vi "Load Instrument Classes.vi"(8 "error in (no error)":errorcluster, 11 "C.E.":refnum<class "Control Experiment.lvclass">) -> (0 "error out":errorcluster, 3 "Control Experiment":refnum<class "Control Experiment.lvclass">)   [LabVIEW 2019, in "Control Experiment.lvclass"]
uses:
  Control Experiment.lvclass
  Typedefs/Instrument Class Rings--Cluster.ctl
  <userlib>/LevyLab/Instrument Framework/Instrument/Instrument.lvclass
  C:/Program Files (x86)/National Instruments/LabVIEW 2019/vi.lib/JKI/JKI SMO/SMO/SMO.lvclass
  Control Experiment.lvclass/Control Experiment.ctl
  Typedefs/Instrument Classes--cluster.ctl
  <userlib>/LevyLab/Instrument Framework/Instrument Types/Lockin/Instrument.LockinAPI.lvclass
  <userlib>/LevyLab/Instrument Framework/Instrument Types/Amplifier/Instrument.Amplifier.lvclass
  <userlib>/LevyLab/Instrument Framework/Instrument Types/Cryostat/Instrument.Cryostat.lvclass
  <userlib>/LevyLab/Instrument Framework/Instrument Types/CBridge/Instrument.CBridge.lvclass
  <userlib>/LevyLab/Instrument Framework/Instrument Types/Delay Line/Instrument.DelayLine.lvclass
  <userlib>/LevyLab/Instrument Framework/Instrument Types/Strain/Instrument.Strain.lvclass
  <userlib>/LevyLab/Instrument Framework/Instrument Types/VNA/Instrument.VNA.lvclass
  <userlib>/LevyLab/Instrument Framework/Instrument Types/VSource/Instrument.VSource.lvclass
  Typedefs/Instrument Types--enum.ctl
  <userlib>/LevyLab/Instrument Framework/Instrument/Instrument.lvclass/Instrument.ctl
  <vilib>/Utility/Data Type/NI_Data Type.lvlib
  Attributes/Instrument Attributes.lvlib
  <vilib>/JKI/JKI SMO/URI Parsing/URI.lvlib
panel:
  in  "DAQ":refnum<visa-resource-name>
  in  "Instrument Addresses":T1 caption="Instruments"
  in  "OK":bool
  in  "Instrument Classes":T2 {"Amplifier" items=["", "Krohn-Hite-7008"]; "DAQ" items=["", "Lockin"]; "Strain Cell" items=["", "RP100"]; "Capacitance" items=["", "AH2500"]; "Level" items=["", "Cryostation", "OxfordVRM", "OptiCool", "PPMS", "PPMS1", "PPMS2", "PPMS3"]; "Rotator" items=["", "Cryostation", "OxfordVRM", "OptiCool", "PPMS", "PPMS1", "PPMS2", "PPMS3"]; "Magnet" items=["", "Cryostation", "OxfordVRM", "OptiCool", "PPMS", "PPMS1", "PPMS2", "PPMS3"]; "Temperature" items=["", "Cryostation", "OxfordVRM", "OptiCool", "PPMS", "PPMS1", "PPMS2", "PPMS3"]}
  out "Status":string
  # "1. Choose / Confirm Instrument Classes"
  # "2. Choose / Confirm Remote Instruments"
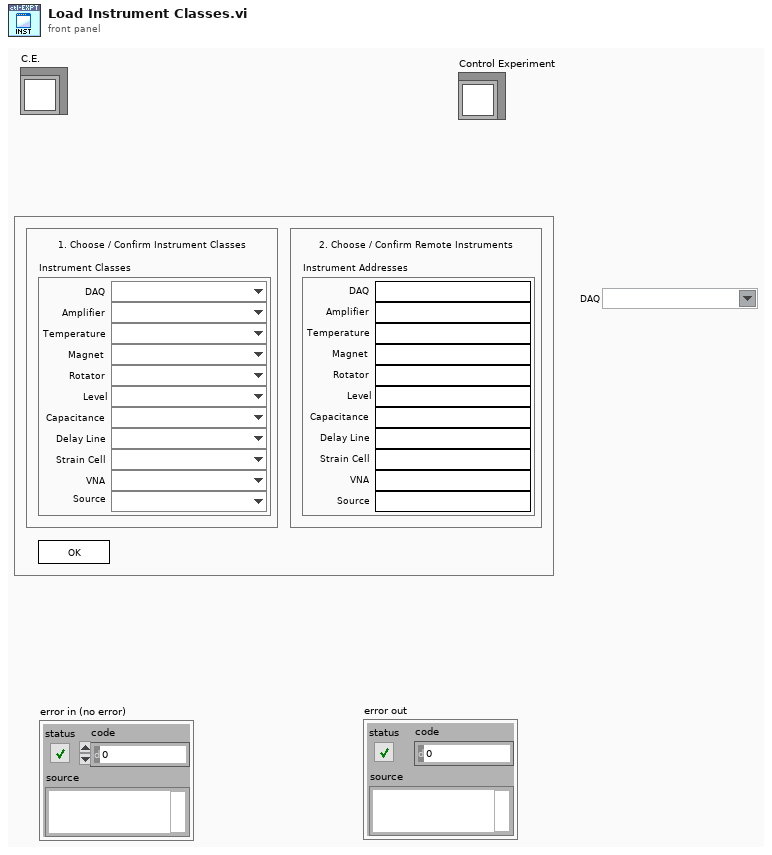
[diagram p1: front panel]
types:
  T1 = cluster{"DAQ":string, "Amplifier":string, "Temperature":string, "Magnet":string, "Rotator":string, "Level":string, "Capacitance Bridge":string, "Delay Line":string, "Strain Cell":string, "VNA":string, "Source":string}
  T2 = typedef "Control Experiment.lvclass/Instrument Class Rings--Cluster.ctl" = cluster{"DAQ":u16, "Amplifier":u16, "Temperature":u16, "Magnet":u16, "Rotator":u16, "Level":u16, "Capacitance":u16, "Delay Line":u16, "Strain Cell":u16, "VNA":u16, "Source":u16}
  T3 = enum32{"Invalid", "Standard", "Closed", "Hidden", "Minimized", "Maximized"}
  T4 = enum32{"invalid app kind", "Development System", "Run Time System", "Student Edition", "Embedded LabVIEW", "Evaluation", "Custom"}
  T5 = typedef "Control Experiment.lvclass/Instrument Classes--cluster.ctl" = cluster{"DAQ":refnum<class "Instrument.LockinAPI.lvclass">, "Amplifier":refnum<class "Instrument.Amplifier.lvclass">, "Temperature":refnum<class "Instrument.Cryostat.lvclass">, "Magnet":refnum<class "Instrument.Cryostat.lvclass">, "Rotator":refnum<class "Instrument.Cryostat.lvclass">, "Level":refnum<class "Instrument.Cryostat.lvclass">, "Capacitance":refnum<class "Instrument.CBridge.lvclass">, "Delay Line":refnum<class "Instrument.DelayLine.lvclass">, "Strain Cell":refnum<class "Instrument.Strain.lvclass">, "VNA":refnum<class "Instrument.VNA.lvclass">, "Source":refnum<class "Instrument.VSource.lvclass">}
  T6 = typedef "Control Experiment.lvclass/Instrument Types--enum.ctl" = enum16{"DAQ", "Amplifier", "Temperature", "Magnet", "Rotator", "Level", "Capacitance", "Delay Line", "Strain Cell", "VNA", "Source"}
  T7 = cluster{"Core":cluster{"Current VI Reference":refnum<vi>, "Close Panel on Exit?":bool}, "C.E.":refnum<class "Control Experiment.lvclass">, "Instruments":refnum<vi>, "Addresses":refnum<vi>, "Instrument Class Rings":refnum<vi>[], "Installed Instruments":refnum<class "Instrument.lvclass">[], "Cast Instruments":refnum<class "Instrument.lvclass">[]}
  T8 = cluster{"Current VI Reference":refnum<vi>, "Close Panel on Exit?":bool}
  T9 = enum32{"Bad", "Idle", "Run top level", "Running"}
  T10 = typedef "Control Experiment.lvclass/Instruments--cluster.ctl" = cluster{"class path":path, "Address":string, "Type":T6}
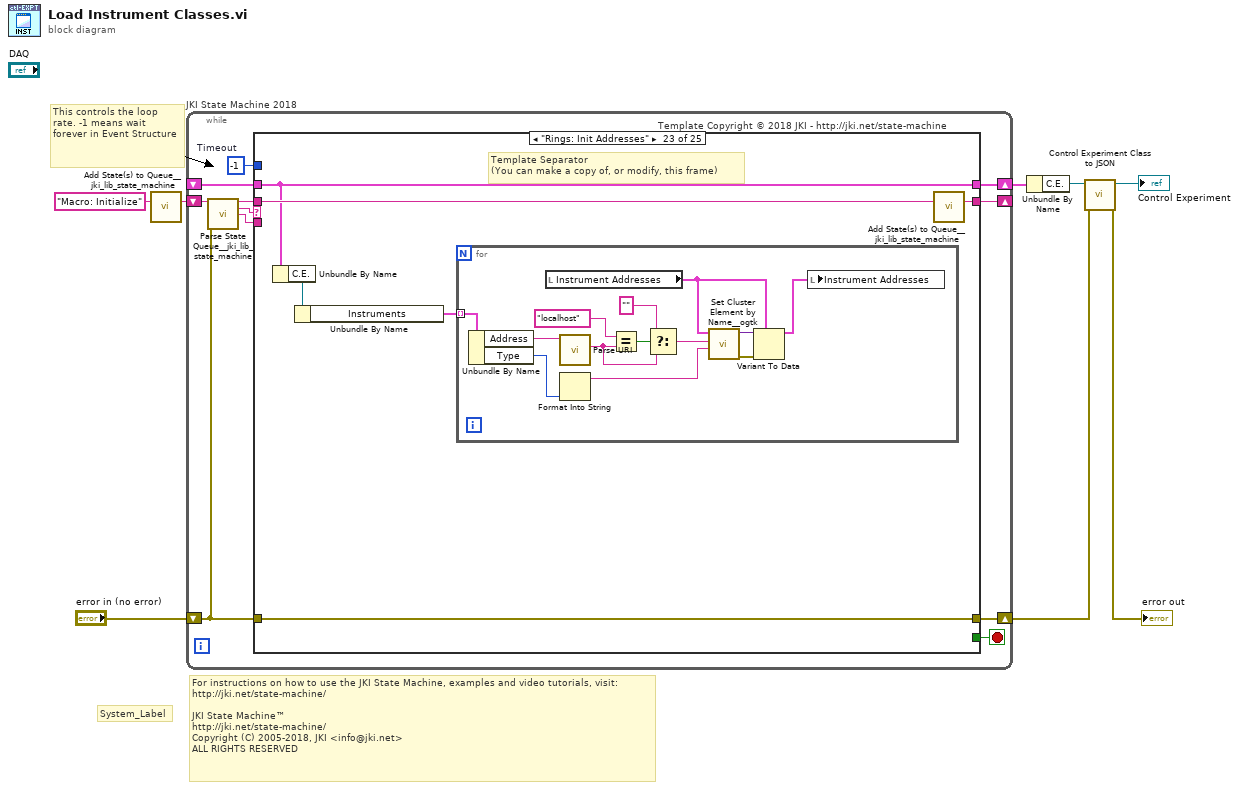
[diagram p0: block diagram]
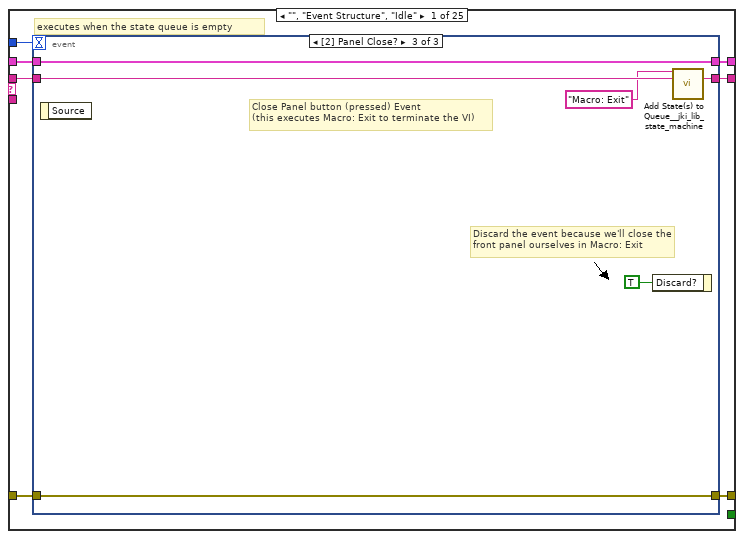
[diagram p2: hidden frame]
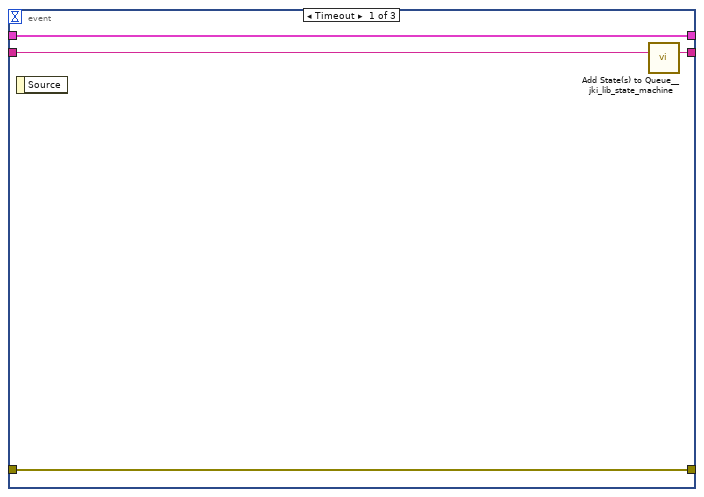
[diagram p3: hidden frame]
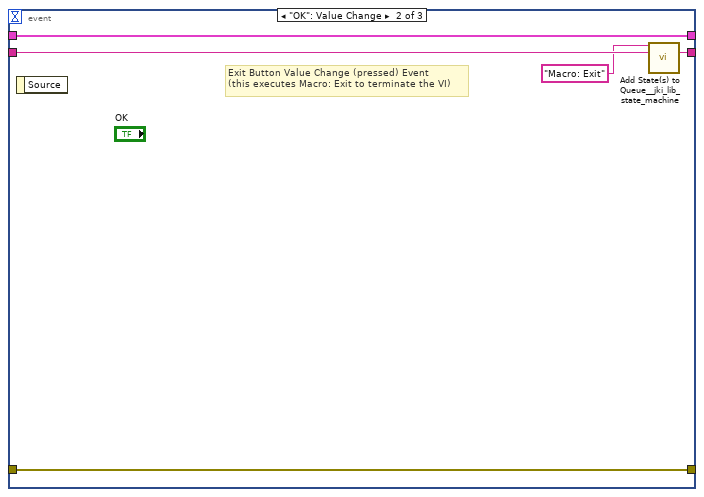
[diagram p4: hidden frame]
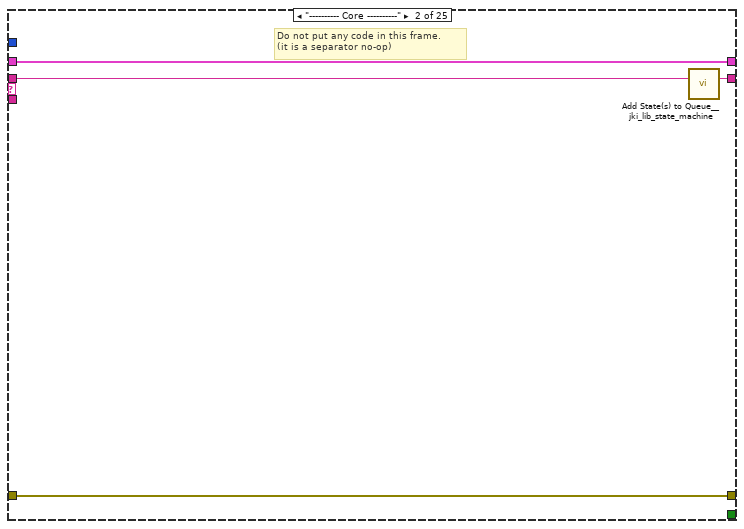
[diagram p5: hidden frame]
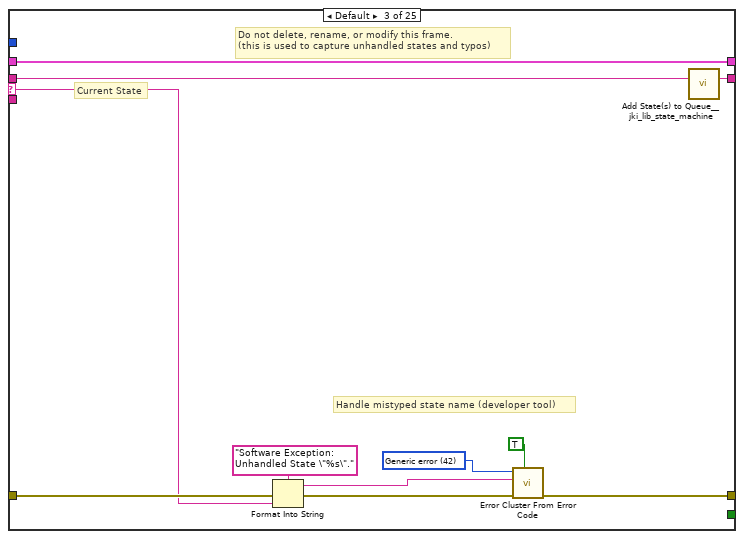
[diagram p6: hidden frame]
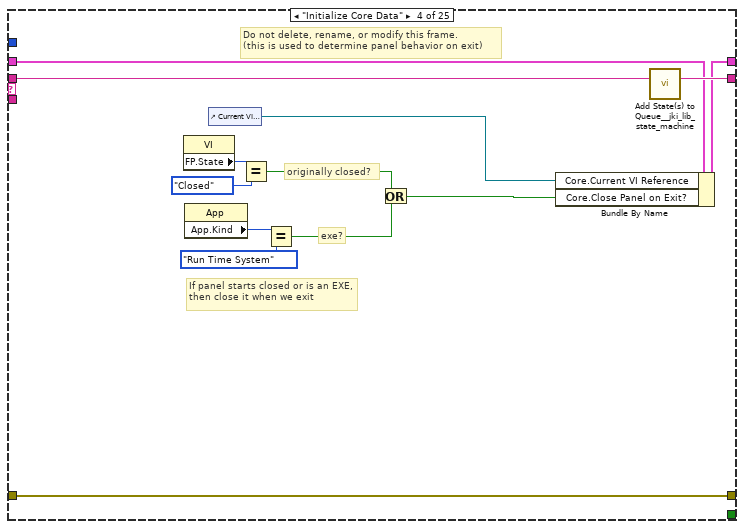
[diagram p7: hidden frame]
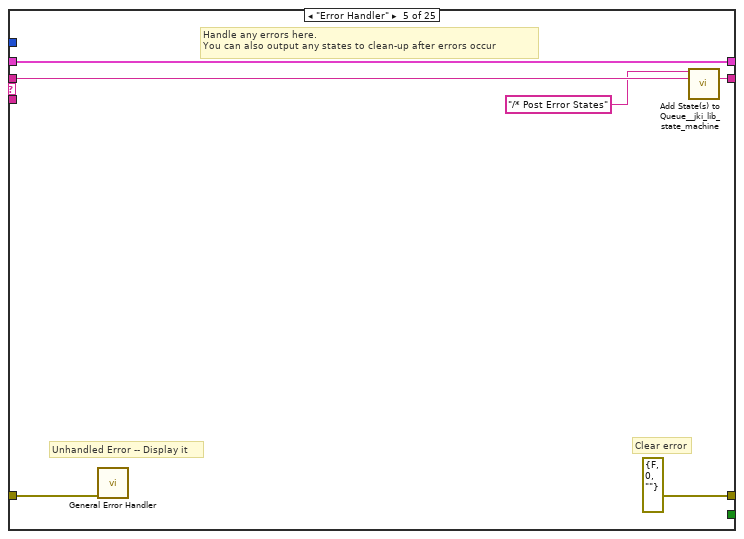
[diagram p8: hidden frame]
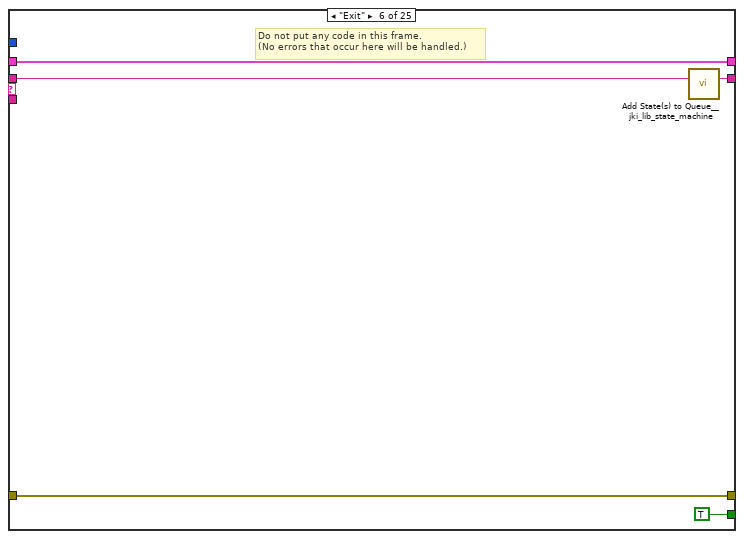
[diagram p9: hidden frame]
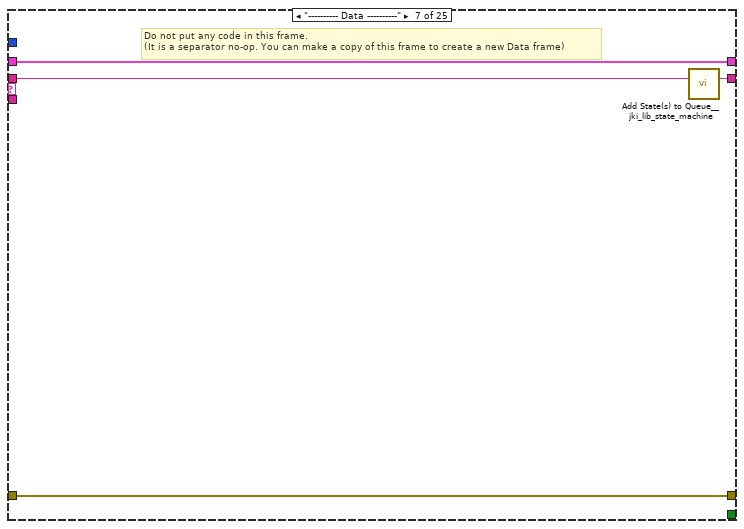
[diagram p10: hidden frame]
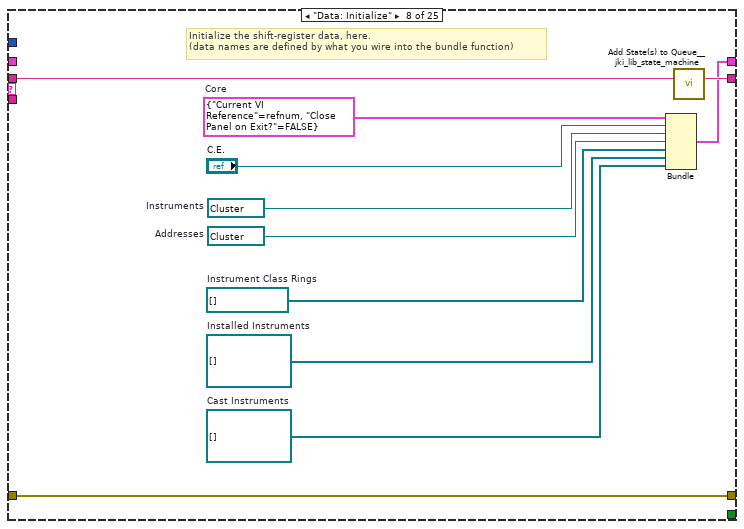
[diagram p11: hidden frame]
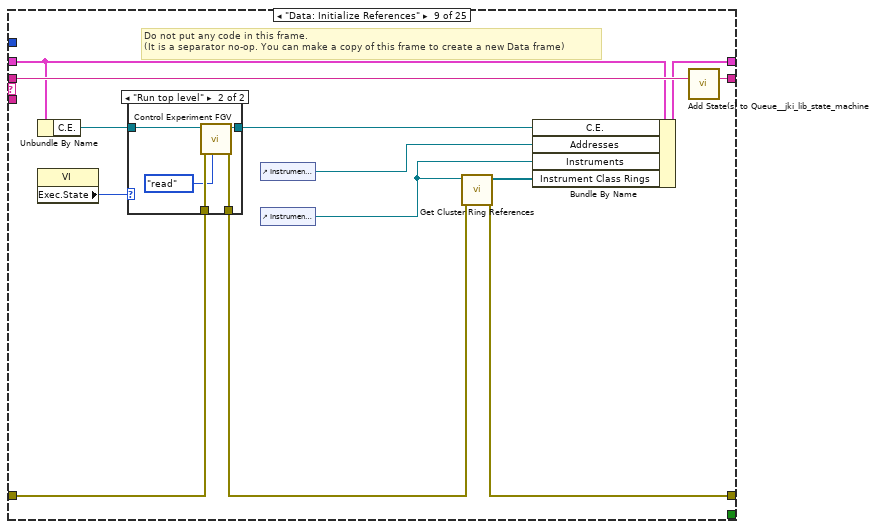
[diagram p12: hidden frame]
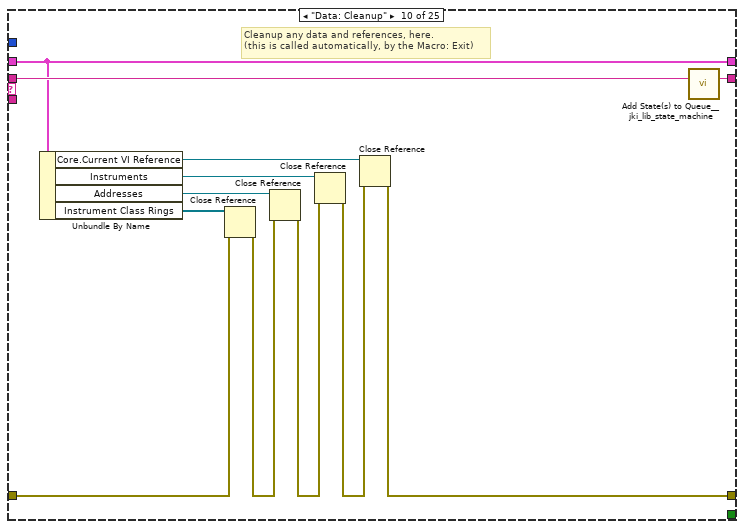
[diagram p14: hidden frame]
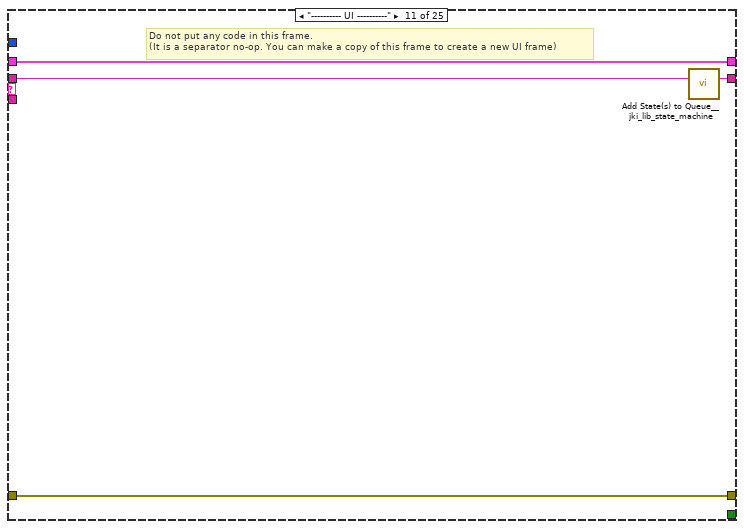
[diagram p15: hidden frame]
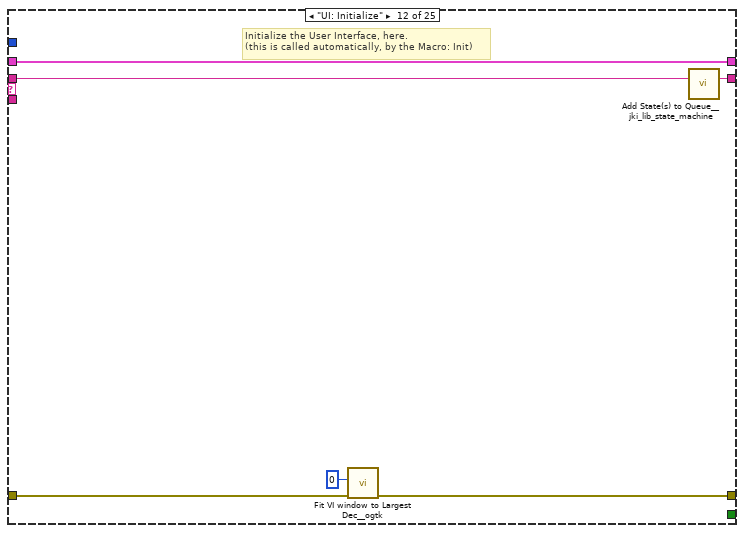
[diagram p16: hidden frame]
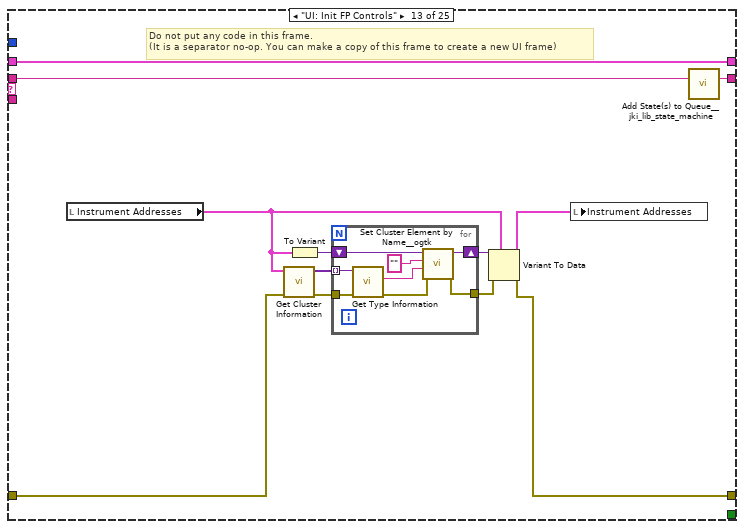
[diagram p17: hidden frame]
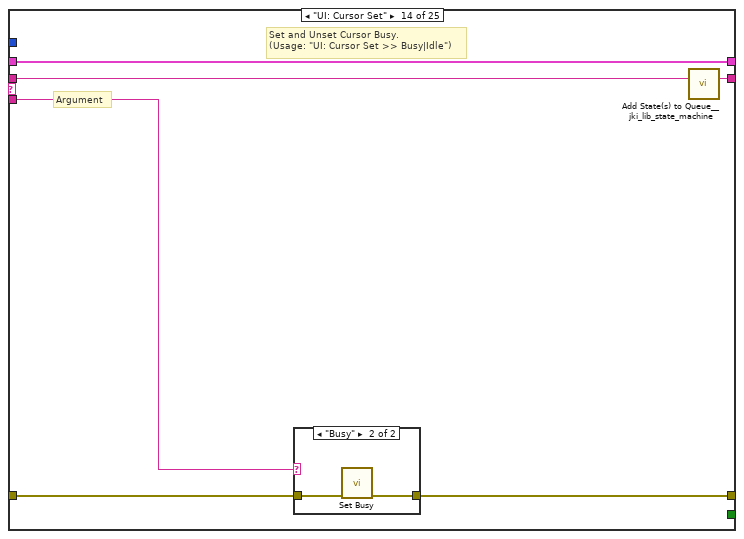
[diagram p18: hidden frame]
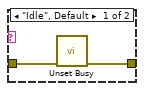
[diagram p19: hidden frame]
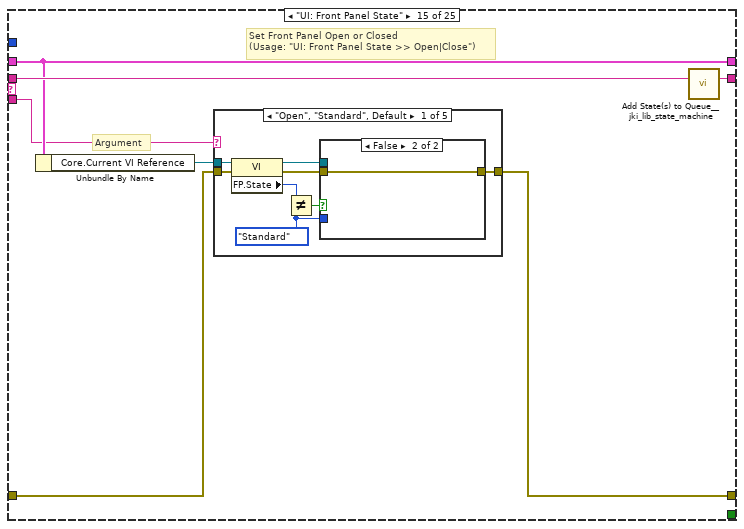
[diagram p20: hidden frame]
diagram:
  # "For instructions on how to use the JKI State Machine, examples and video tutorials, visit:\nhttp://jki.net/state-machine/\n\nJKI State Machine™\nhttp://jki.net/state-machine/\nCopyright (C) 2005-2018, JKI <info@jki.net>\nALL RIGHTS RESERVED"
  # "This controls the loop rate. -1 means wait forever in Event Structure"
  # "System_Label"
  n1 = call <vilib>:"Add State(s) to Queue__jki_lib_state_machine.vi"("State(s) in (\"\")"="Macro: Initialize") -> ("States Out"=w8:string)  [unwired: 14 in]
  n2 = while "JKI State Machine 2018" {
    shift-right: [w12] -> w6
    shift-left: _ -> [w11]
    shift-right: [w15] -> w2
    shift-left: "error in (no error)" -> [w9]
    shift-right: [w14] -> _
    shift-left: w8 -> [w16]
    stop <- w13 stop-if-true
    w10 = -1  # Timeout
    # "Template Copyright © 2018 JKI - http://jki.net/state-machine"
    n3 = call <vilib>:"Parse State Queue__jki_lib_state_machine.vi"("State Queue"=w16, "Error In (no error)"=w9) -> ("Remaining States"=w18:string, "Current State"=w19:string, "Arguments"=w17:string)  [unwired: 11 in]
    n4 = case shown="\"Rings: Init Addresses\"" w19 {
      selector: w19 -> [_ _ w46 _ _ _ _ _ _ _ _ _ _ _ _ _ _ _ _ _ _ _ _ _ _]
      tunnel: w18 -> [w26 w45 w50 w69 w75 w80 w84 w95 w108 w127 w131 w137 w149 w163 w174 w243 w248 w259 w263 w269 w282 w303 w309 w326 w342]
      tunnel: w17 -> [_ _ _ _ _ _ _ _ _ _ _ _ _ w158 w168 _ _ _ _ _ _ _ _ _ _]
      tunnel: w11 -> [w24 w42 w48 w62 w72 w78 w81 _ w101 w123 w128 w133 w143 w161 w170 w240 w245 w256 w260 w266 w275 w296 w306 w323 w336]
      tunnel: [w23 w43 w52 w66 errorcluster {"status"=FALSE, "code"=0, "source"=""} ("error out") w77 w82 w92 w104 w124 w129 w135 w140 w159 w171 w241 w246 w257 w261 w265 w274 w301 w307 w324 w338] -> w15
      tunnel: w9 -> [w22 w43 w51 w66 w71 w77 w82 w92 w102 w119 w129 w134 w139 w160 w172 w241 w246 w257 w261 w264 w274 w300 w307 w324 w328]
      tunnel: [w25 w44 w49 w68 w74 w79 w83 w94 w107 w126 w130 w136 w148 w162 w173 w242 w247 w258 w262 w268 w281 w302 w308 w325 w341] -> w14
      tunnel: [_ _ _ _ _ TRUE _ _ _ _ _ _ _ _ _ _ _ _ _ _ _ _ _ _ _] -> w13
      tunnel: [w21 w42 w48 w67 w72 w78 w81 w93 w106 w123 w128 w133 w143 w161 w170 w240 w245 w256 w260 w266 w276 w296 w306 w323 w337] -> w12
      tunnel: w10 -> [w20 _ _ _ _ _ _ _ _ _ _ _ _ _ _ _ _ _ _ _ _ _ _ _ _]
      frame "", "Event Structure", "Idle" {
        # "executes when the state queue is empty"
        n5 = event shown="[2] Panel Close?" {
          selector: _ -> [_ _ _]
          dyn-events: _ -> [_ _ _]
          timeout: w20 -> [_ _ _]
          tunnel: w26 -> [w30 w35 w41]
          tunnel: [w29 w34 w40] -> w25
          tunnel: w24 -> [w27 w32 w38]
          tunnel: [w28 w33 w39] -> w23
          tunnel: w22 -> [w28 w33 w39]
          tunnel: [w27 w32 w38] -> w21
          event Timeout {
            n6 = event-data() -> ()  [unwired: 1 in, 1 out]
            n7 = call <vilib>:"Add State(s) to Queue__jki_lib_state_machine.vi"("State(s) in (\"\")"=w30) -> ("States Out"=w29:string)  [unwired: 14 in]
          }
          event "OK": Value Change {
            # "Exit Button Value Change (pressed) Event\n(this executes Macro: Exit to terminate the VI)"
            n8 = event-data() -> ()  [unwired: 1 in, 1 out]
            n9 = call <vilib>:"Add State(s) to Queue__jki_lib_state_machine.vi"("State(s) in Front (\"\")"="Macro: Exit", "State(s) in (\"\")"=w35) -> ("States Out"=w34:string)  [unwired: 13 in]
          }
          event Panel Close? {
            # "Discard the event because we'll close the front panel ourselves in Macro: Exit"
            # "Close Panel button (pressed) Event\n(this executes Macro: Exit to terminate the VI)"
            n10 = event-data() -> ()  [unwired: 1 in, 1 out]
            n11 = event-data("Discard?"=TRUE) -> ()  [unwired: 1 in, 1 out]
            n12 = call <vilib>:"Add State(s) to Queue__jki_lib_state_machine.vi"("State(s) in Front (\"\")"="Macro: Exit", "State(s) in (\"\")"=w41) -> ("States Out"=w40:string)  [unwired: 13 in]
          }
        }
      }
      frame "---------- Core ----------" {
        # "Do not put any code in this frame.\n(it is a separator no-op)"
        n13 = call <vilib>:"Add State(s) to Queue__jki_lib_state_machine.vi"("State(s) in (\"\")"=w45) -> ("States Out"=w44:string)  [unwired: 14 in]
      }
      frame Default {
        w55 = 42 items=["No error", "Argument error", "Memory is full", "Out of zone", "End of file", "File already open", "Generic file I/O error", "File not found", "File permission error", "Disk is full", "Duplicate path", "Too many files open", "System feature not enabled", "Resource file not found", "Cannot add resource", "Resource not found", "Image not found", "Image memory error", "Pen does not exist", "Config type invalid", "Config token not found", "Config parse error", "Config memory error", "Bad external code format", "Bad external code offset", "External code not present", "Null window", "Destroy window error", "Null menu", "Print aborted", "Bad print record", "Print driver error", "Windows error during printing", "Memory error during printing", "Print dialog error", "Generic print error", "Invalid device refnum", "Device not found", "Device parameter error", "Device unit error", "Cannot open device", "Device call aborted", "Generic error", "Cancelled by user", "Object ID too low", "Object ID too high", "Object not in heap", "Unknown heap", "Unknown object (invalid DefProc)", "Unknown object (DefProc not in table)", "Message out of range", "Invalid (null) method", "Unknown message", "Manager call not supported", "Bad address", "Network operation in progress", "Network operation timed out", "Connection is busy", "Network attribute not supported", "Network error", "Address in use", "System out of memory", "Connection aborted", "Connection refused", "Not connected", "Already connected", "Connection closed", "Initialization error (interapplication manager)", "Bad occurrence", "Wait on unbound occurrence handler", "Occurrence queue overflow", "Datalog type conflict", "Unused", "Unrecognized type (interapplication manager)", "Memory corrupt", "Failed to make temporary DLL", "Old CIN version", "Drag socket not found", "Failed to load drop-object", "Failed to register OLE object", "Failed to release OLE object", "Format specifier type mismatch", "Unknown format specifier", "Too few format specifiers", "Too many format specifiers", "Scan failed", "Newer CIN version", "Error converting to variant", "Runtime menu error", "Password tampered", "Variant attribute not found", "Incompatible variant data type", "Event data is not available", "Event Store is not present", "Occurrence is not found", "Event Queue is not created", "Event info is not available", "Refnum passed is NULL", "Error retrieving Class GUID", "Error retrieving CoClass GUID", "Error retrieving TypeLib GUID.", "Bad built application magic bytes.", "Specific driver is different from the specific driver associated with the Logical Name.", "There is no session opened to the class driver.", "Max Error", "MAX - Error with config objects", "MAX - Error loading configuration", "MAX - Group not supported"]
        # "Current State"
        # "Do not delete, rename, or modify this frame.\n(this is used to capture unhandled states and typos)"
        # "Handle mistyped state name (developer tool)"
        n14 = Format Into String(format string="Software Exception: Unhandled State \"%s\"." ("message"), error in=w51, w46) -> (resulting string=w54:string, error out=w53:errorcluster)  [unwired: 1 in]
        n15 = call <vilib>:"Error Cluster From Error Code.vi"("show call chain? (False)"=TRUE, "error in (no error)"=w53, "error message (\"\")"=w54, "error code (0)"=w55) -> ("error out"=w52:errorcluster)  [unwired: 5 in]
        n16 = call <vilib>:"Add State(s) to Queue__jki_lib_state_machine.vi"("State(s) in (\"\")"=w50) -> ("States Out"=w49:string)  [unwired: 14 in]
      }
      frame "Initialize Core Data" {
        # "Do not delete, rename, or modify this frame.\n(this is used to determine panel behavior on exit)"
        # "originally closed?"
        # "exe?"
        # "If panel starts closed or is an EXE, then close it when we exit"
        n17 = property class="VI"() -> ("FP.State"=w59:T3)  [unwired: 2 in, 2 out]
        n18 = property class="App"() -> ("App.Kind"=w65:T4)  [unwired: 2 in, 2 out]
        n19 = control-ref of="Current VI Reference"() -> (w60:refnum<vi>)
        n20 = Equal?(x=w59, y=T3."Closed" ("Front Panel Window:State")) -> (x = y?=w57:bool)
        n21 = Equal?(x=w65, y=T4."Run Time System" ("Application:Kind")) -> (x = y?=w63:bool)
        n22 = Or(x=w57, y=w63) -> (x .or. y?=w61:bool)
        n23 = Bundle By Name(cluster=w62, "Core.Current VI Reference"=w60, "Core.Close Panel on Exit?"=w61) -> (w67:T7)
        n24 = call <vilib>:"Add State(s) to Queue__jki_lib_state_machine.vi"("State(s) in (\"\")"=w69) -> ("States Out"=w68:string)  [unwired: 14 in]
      }
      frame "Error Handler" {
        # "Unhandled Error -- Display it"
        # "Handle any errors here.\nYou can also output any states to clean-up after errors occur"
        # "Clear error"
        n25 = call <vilib>:"General Error Handler.vi"("error in (no error)"=w71) -> ()  [unwired: 10 in, 5 out]
        n26 = call <vilib>:"Add State(s) to Queue__jki_lib_state_machine.vi"("State(s) in Front (\"\")"="/* Post Error States", "State(s) in (\"\")"=w75) -> ("States Out"=w74:string)  [unwired: 13 in]
      }
      frame "Exit" {
        # "Do not put any code in this frame.\n(No errors that occur here will be handled.)"
        n27 = call <vilib>:"Add State(s) to Queue__jki_lib_state_machine.vi"("State(s) in (\"\")"=w80) -> ("States Out"=w79:string)  [unwired: 14 in]
      }
      frame "---------- Data ----------" {
        # "Do not put any code in this frame.\n(It is a separator no-op. You can make a copy of this frame to create a new Data frame)"
        n28 = call <vilib>:"Add State(s) to Queue__jki_lib_state_machine.vi"("State(s) in (\"\")"=w84) -> ("States Out"=w83:string)  [unwired: 14 in]
      }
      frame "Data: Initialize" {
        w85 = refnum<vi> refnum  # Addresses
        w87 = refnum<vi> refnum  # Instruments
        w88 = refnum<class "Instrument.lvclass">[] []  # Cast Instruments
        w89 = refnum<vi>[] []  # Instrument Class Rings
        w90 = refnum<class "Instrument.lvclass">[] []  # Installed Instruments
        w91 = T8 {"Current VI Reference"=refnum, "Close Panel on Exit?"=FALSE}  # Core
        # "Initialize the shift-register data, here.\n(data names are defined by what you wire into the bundle function)"
        n29 = Bundle("Core"=w91, "C.E."="C.E.", "Instruments"=w87, "Addresses"=w85, "Instrument Class Rings"=w89, "Installed Instruments"=w90, "Cast Instruments"=w88) -> (w93:T7)  [unwired: 1 in]
        n30 = call <vilib>:"Add State(s) to Queue__jki_lib_state_machine.vi"("State(s) in (\"\")"=w95) -> ("States Out"=w94:string)  [unwired: 14 in]
      }
      frame "Data: Initialize References" {
        # "Do not put any code in this frame.\n(It is a separator no-op. You can make a copy of this frame to create a new Data frame)"
        n31 = Unbundle By Name(w101) -> ("C.E."=w100:refnum<class "Control Experiment.lvclass">)
        n32 = property class="VI"() -> ("Exec.State"=w99:T9)  [unwired: 2 in, 2 out]
        n33 = case shown="\"Run top level\"" w99 {
          tunnel: [w109 w115] -> w103
          tunnel: w102 -> [w109 w114]
          tunnel: [w110 w112] -> w97
          tunnel: w100 -> [w110 w111]
          frame Default {
          }
          frame "Run top level" {
            n34 = call "Control Experiment FGV.vi"("Function"=enum16{"read", "write"}."read", "error in (no error)"=w114, "Control Experiment.lvclass"=w111) -> ("error out"=w115:errorcluster, "Control Experiment.lvclass out"=w112:refnum<class "Control Experiment.lvclass">)  [unwired: 7 in]
          }
        }
        n35 = control-ref of="Instrument Addresses"() -> (w98:refnum<vi>)
        n36 = control-ref of="Instrument Classes"() -> (w96:refnum<vi>)
        n37 = call "Get Cluster Ring References.vi"("error in (no error)"=w103, "Cluster Reference in"=w96) -> ("error out"=w104:errorcluster, "Ring References"=w105:refnum<vi>[])  [unwired: 8 in]
        n38 = Bundle By Name(cluster=w101, "C.E."=w97, "Addresses"=w98, "Instruments"=w96, "Instrument Class Rings"=w105) -> (w106:T7)
        n39 = call <vilib>:"Add State(s) to Queue__jki_lib_state_machine.vi"("State(s) in (\"\")"=w108) -> ("States Out"=w107:string)  [unwired: 14 in]
      }
      frame "Data: Cleanup" {
        # "Cleanup any data and references, here.\n(this is called automatically, by the Macro: Exit)"
        n40 = Unbundle By Name(w123) -> ("Core.Current VI Reference"=w125:refnum<vi>, "Instruments"=w122:refnum<vi>, "Addresses"=w121:refnum<vi>, "Instrument Class Rings"=w120:refnum<vi>[])
        n41 = Close Reference(reference=w120, error in (no error)=w119) -> (error out=w118:errorcluster)
        n42 = Close Reference(reference=w121, error in (no error)=w118) -> (error out=w117:errorcluster)
        n43 = Close Reference(reference=w122, error in (no error)=w117) -> (error out=w116:errorcluster)
        n44 = Close Reference(reference=w125, error in (no error)=w116) -> (error out=w124:errorcluster)
        n45 = call <vilib>:"Add State(s) to Queue__jki_lib_state_machine.vi"("State(s) in (\"\")"=w127) -> ("States Out"=w126:string)  [unwired: 14 in]
      }
      frame "---------- UI ----------" {
        # "Do not put any code in this frame.\n(It is a separator no-op. You can make a copy of this frame to create a new UI frame)"
        n46 = call <vilib>:"Add State(s) to Queue__jki_lib_state_machine.vi"("State(s) in (\"\")"=w131) -> ("States Out"=w130:string)  [unwired: 14 in]
      }
      frame "UI: Initialize" {
        # "Initialize the User Interface, here.\n(this is called automatically, by the Macro: Init)"
        n47 = call <userlib>:"Fit VI window to Largest Dec__ogtk.vi"("error in (no error)"=w134, "border spacing (2 px)"=0) -> ("error out"=w135:errorcluster)  [unwired: 4 in, 1 out]
        n48 = call <vilib>:"Add State(s) to Queue__jki_lib_state_machine.vi"("State(s) in (\"\")"=w137) -> ("States Out"=w136:string)  [unwired: 14 in]
      }
      frame "UI: Init FP Controls" {
        # "Do not put any code in this frame.\n(It is a separator no-op. You can make a copy of this frame to create a new UI frame)"
        n49 = local read "Instrument Addresses"() -> (w138:T1)
        n50 = call <vilib>:"Get Cluster Information.vi"("error in (no error)"=w139, "variant"=w138) -> ("error out"=w145:errorcluster, "cluster elements"=w147:variant[])  [unwired: 8 in]
        n51 = To Variant(anything=w138) -> (Variant=w142:variant)
        n52 = for {
          tunnel: w147 -> [w157] mode=indexing
          shift-right: [w155] -> w146
          shift-left: w142 -> [w156]
          tunnel: w145 -> [w150]
          tunnel: [w151] -> w144
          n53 = call <vilib>:"Get Type Information.vi"("error in (no error)"=w150, "variant"=w157) -> ("error out"=w152:errorcluster, "name"=w153:string)  [unwired: 5 in, 3 out]
          n54 = call <userlib>:"Set Cluster Element by Name__ogtk.vi"("error in (no error)"=w152, "Element Name (\"\": New Element Data Name)"=w153, "New Element Value"="", "Cluster"=w156) -> ("error out"=w151:errorcluster, "VCluster out"=w155:variant)  [unwired: 5 in, 1 out]
        }
        n55 = Variant To Data(error in=w144, type=w138, Variant=w146) -> (data=w141:T1, error out=w140:errorcluster)
        n56 = local write "Instrument Addresses"(w141) -> ()
        n57 = call <vilib>:"Add State(s) to Queue__jki_lib_state_machine.vi"("State(s) in (\"\")"=w149) -> ("States Out"=w148:string)  [unwired: 14 in]
      }
      frame "UI: Cursor Set" {
        # "Argument"
        # "Set and Unset Cursor Busy.\n(Usage: \"UI: Cursor Set >> Busy|Idle\")"
        n58 = case shown="\"Busy\"" w158 {
          tunnel: w160 -> [w165 w167]
          tunnel: [w164 w166] -> w159
          frame "Idle", Default {
            n59 = call <vilib>:"Unset Busy.vi"("error in (no error)"=w165) -> ("error out"=w164:errorcluster)  [unwired: 10 in]
          }
          frame "Busy" {
            n60 = call <vilib>:"Set Busy.vi"("error in (no error)"=w167) -> ("error out"=w166:errorcluster)  [unwired: 9 in, 1 out]
          }
        }
        n61 = call <vilib>:"Add State(s) to Queue__jki_lib_state_machine.vi"("State(s) in (\"\")"=w163) -> ("States Out"=w162:string)  [unwired: 14 in]
      }
      frame "UI: Front Panel State" {
        # "Argument"
        # "Set Front Panel Open or Closed\n(Usage: \"UI: Front Panel State >> Open|Close\")"
        n62 = Unbundle By Name(w170) -> ("Core.Current VI Reference"=w169:refnum<vi>)
        n63 = case shown="\"Open\", \"Standard\", Default" w168 {
          tunnel: w172 -> [w180 w195 w206 w219 w232]
          tunnel: [w182 w196 w208 w221 w234] -> w171
          tunnel: w169 -> [w181 w193 w207 w220 w233]
          frame "Open", "Standard", Default {
            w175 = T3."Standard" ("State")
            n64 = property class="VI"(reference=w181, error in=w180) -> (reference out=w178:refnum<vi>, error out=w179:errorcluster, "FP.State"=w177:T3)
            n65 = Not Equal?(x=w177, y=w175) -> (x != y?=w176:bool)
            n66 = case shown="False" w176 {
              tunnel: [w186 w188] -> w182
              tunnel: w179 -> [w185 w188]
              tunnel: w178 -> [w184 _]
              tunnel: w175 -> [w183 _]
              frame True {
                n67 = invoke class="VI" method="FP.Open"(reference=w184, error in=w185, "Activate"=TRUE, "State"=w183) -> (error out=w186:errorcluster)  [unwired: 1 in, 4 out]
              }
              frame False {
              }
            }
          }
          frame "Close", "Closed" {
            n68 = property class="VI"(reference=w193, error in=w195) -> (reference out=w192:refnum<vi>, error out=w194:errorcluster, "FP.State"=w190:T3)
            n69 = Not Equal?(x=w190, y=T3."Closed" ("Front Panel Window:State")) -> (x != y?=w189:bool)
            n70 = case shown="True" w189 {
              tunnel: [w197 w200] -> w196
              tunnel: w194 -> [w197 w199]
              tunnel: w192 -> [_ w198]
              frame False {
              }
              frame True {
                n71 = invoke class="VI" method="FP.Close"(reference=w198, error in=w199) -> (error out=w200:errorcluster)  [unwired: 1 in, 2 out]
              }
            }
          }
          frame "Hidden", "Hide" {
            w201 = T3."Hidden" ("State")
            n72 = property class="VI"(reference=w207, error in=w206) -> (reference out=w204:refnum<vi>, error out=w205:errorcluster, "FP.State"=w203:T3)
            n73 = Not Equal?(x=w203, y=w201) -> (x != y?=w202:bool)
            n74 = case shown="True" w202 {
              tunnel: [w212 w213] -> w208
              tunnel: w205 -> [w211 w213]
              tunnel: w204 -> [w210 _]
              tunnel: w201 -> [w209 _]
              frame True {
                n75 = invoke class="VI" method="FP.Open"(reference=w210, error in=w211, "State"=w209) -> (error out=w212:errorcluster)  [unwired: 2 in, 4 out]
              }
              frame False {
              }
            }
          }
          frame "Minimize", "Minimized" {
            w214 = T3."Minimized" ("State")
            n76 = property class="VI"(reference=w220, error in=w219) -> (reference out=w217:refnum<vi>, error out=w218:errorcluster, "FP.State"=w216:T3)
            n77 = Not Equal?(x=w216, y=w214) -> (x != y?=w215:bool)
            n78 = case shown="True" w215 {
              tunnel: [w225 w226] -> w221
              tunnel: w218 -> [w224 w226]
              tunnel: w217 -> [w223 _]
              tunnel: w214 -> [w222 _]
              frame True {
                n79 = invoke class="VI" method="FP.Open"(reference=w223, error in=w224, "State"=w222) -> (error out=w225:errorcluster)  [unwired: 2 in, 4 out]
              }
              frame False {
              }
            }
          }
          frame "Maximize", "Maximized" {
            w227 = T3."Maximized" ("State")
            n80 = property class="VI"(reference=w233, error in=w232) -> (reference out=w230:refnum<vi>, error out=w231:errorcluster, "FP.State"=w229:T3)
            n81 = Not Equal?(x=w229, y=w227) -> (x != y?=w228:bool)
            n82 = case shown="True" w228 {
              tunnel: [w238 w239] -> w234
              tunnel: w231 -> [w237 w239]
              tunnel: w230 -> [w236 _]
              tunnel: w227 -> [w235 _]
              frame True {
                n83 = invoke class="VI" method="FP.Open"(reference=w236, error in=w237, "State"=w235) -> (error out=w238:errorcluster)  [unwired: 2 in, 4 out]
              }
              frame False {
              }
            }
          }
        }
        n84 = call <vilib>:"Add State(s) to Queue__jki_lib_state_machine.vi"("State(s) in (\"\")"=w174) -> ("States Out"=w173:string)  [unwired: 14 in]
      }
      frame "---------- Macro ----------" {
        # "Do not put any code in this frame.\n(It is a separator no-op. You can make a copy of this frame to create a new Macro frame)"
        n85 = call <vilib>:"Add State(s) to Queue__jki_lib_state_machine.vi"("State(s) in (\"\")"=w243) -> ("States Out"=w242:string)  [unwired: 14 in]
      }
      frame "Macro: Initialize" {
        # "Initialization Macro\n(This is called once, when the VI starts)"
        n86 = call <vilib>:"Add State(s) to Queue__jki_lib_state_machine.vi"("State(s) in Front (\"\")"="Data: Initialize\nInitialize Core Data\nUI: Initialize\nUI: Front Panel State >> Open\n\nData: Initialize References\nUI: Init FP Controls\n\nRings: Empty Rings\nRings: List Installed\nRings: Installed to Rings\n\nRings: Init Addresses", "State(s) in (\"\")"=w248) -> ("States Out"=w247:string)  [unwired: 13 in]
      }
      frame "Macro: Exit" {
        # "Exit Macro\n(This is called once, when the VI exits)"
        n87 = Unbundle By Name(w256) -> ("Core.Close Panel on Exit?"=w255:bool)
        n88 = Select(t="UI: Front Panel State >> Close", s=w255, f="") -> (s? t:f=w252:string)
        n89 = call <vilib>:"Add State(s) to Queue__jki_lib_state_machine.vi"("State(s) in Front (\"\")"="Instruments: Init Instruments" ("State(s) in Front (\"\")"), "State(s) in (\"\")"=w252, "State(s) at Back (\"\")"="Data: Cleanup\nExit") -> ("States Out"=w250:string)  [unwired: 12 in]
        n90 = call <vilib>:"Add State(s) to Queue__jki_lib_state_machine.vi"("State(s) in Front (\"\")"=w250, "State(s) in (\"\")"=w259) -> ("States Out"=w258:string)  [unwired: 13 in]
      }
      frame "---------- Rings ----------" {
        # "Template Separator\n(You can make a copy of, or modify, this frame)"
        n91 = call <vilib>:"Add State(s) to Queue__jki_lib_state_machine.vi"("State(s) in (\"\")"=w263) -> ("States Out"=w262:string)  [unwired: 14 in]
      }
      frame "Rings: Empty Rings" {
        # "Template Separator\n(You can make a copy of, or modify, this frame)"
        n92 = Unbundle By Name(w266) -> ("Instrument Class Rings"=w267:refnum<vi>[])
        n93 = call "Empty Rings.vi"("error in (no error)"=w264, "Ring References"=w267) -> ("error out"=w265:errorcluster)  [unwired: 8 in, 1 out]
        n94 = call <vilib>:"Add State(s) to Queue__jki_lib_state_machine.vi"("State(s) in (\"\")"=w269) -> ("States Out"=w268:string)  [unwired: 14 in]
      }
      frame "Rings: List Installed" {
        # "List all classes in \\user.lib\\LevyLab\n(but not \\user.lib\\LevyLab\\Instrument Framework\\\nor Build Support\\)"
        # "Your code here.\n(You can make a copy of, or modify, this frame)"
        n95 = call "Application user.lib.vi"() -> ("path out"=w271:path)  [unwired: 10 in, 1 out]
        n96 = Build Path(base path=w271, name or relative path="LevyLab") -> (appended path=w270:path)
        n97 = call <vilib>:"Recursive File List.vi"("Folders to Exclude"=string[] ["Instrument Framework", "Build Support"], "pattern"="*.lvclass", "Folder Path"=w270) -> ("All Files in Dir"=w280:path[])  [unwired: 4 in, 4 out]
        n98 = for {
          tunnel: w280 -> [w287] mode=indexing
          tunnel: [w292] -> w273 mode=indexing if=w290
          tunnel: w274 -> [w289]
          tunnel: ["" ("String 2")] -> w272
          # "Find children of Instrument"
          n99 = call <vilib>:"Get LV Class Default Value.vi"("error in (no error)"=w289, "class path"=w287) -> ("error out"=w294:errorcluster, "object"=w295:refnum<class>)  [unwired: 8 in]
          n100 = To More Specific Class(target class=refnum<class "Instrument.lvclass"> refnum ("Instrument"), reference=w295, error in=w294) -> (specific class reference=w292:refnum<class "Instrument.lvclass">, error out=w283:errorcluster)
          n101 = Format Into String(format string="Loading...%s", w287) -> (resulting string=→"Status":string)  [unwired: 2 in, 1 out]
          n102 = Unbundle By Name(w283) -> ("status"=w293:bool)
          n103 = Wait (ms)(milliseconds to wait=u32 5) -> ()  [unwired: 1 out]
          n104 = Not(x=w293) -> (.not. x?=w290:bool)
        }
        n105 = Bundle By Name(cluster=w275, "Installed Instruments"=w273) -> (w276:T7)
        n106 = local write "Status"(w272) -> ()
        n107 = call <vilib>:"Add State(s) to Queue__jki_lib_state_machine.vi"("State(s) in (\"\")"=w282) -> ("States Out"=w281:string)  [unwired: 14 in]
      }
      frame "Rings: Installed to Rings" {
        # "Your code here.\n(You can make a copy of, or modify, this frame)"
        n108 = Unbundle By Name(w296) -> ("C.E."=w299:refnum<class "Control Experiment.lvclass">, "Instrument Class Rings"=w297:refnum<vi>[], "Installed Instruments"=w298:refnum<class "Instrument.lvclass">[])
        n109 = call "Installed Classes to Rings.vi"("error in (no error)"=w300, "Installed"=w298, "Rings"=w297, "C.E."=w299) -> ("error out"=w301:errorcluster)  [unwired: 6 in, 1 out]
        n110 = call <vilib>:"Add State(s) to Queue__jki_lib_state_machine.vi"("State(s) in (\"\")"=w303) -> ("States Out"=w302:string)  [unwired: 14 in]
      }
      frame "Rings: Init Addresses" {
        # "Template Separator\n(You can make a copy of, or modify, this frame)"
        n111 = Unbundle By Name(w306) -> ("C.E."=w304:refnum<class "Control Experiment.lvclass">)
        n112 = Unbundle By Name(w304) -> ("Instruments"=w305:T10[])
        n113 = for {
          tunnel: w305 -> [w322] mode=indexing
          n114 = Unbundle By Name(w322) -> ("Address"=w316:string, "Type"=w318:T6)
          n115 = local read "Instrument Addresses"() -> (w317:T1)
          n116 = call <vilib>:"Parse URI.vi"("URI"=w316) -> ("address"=w310:string)  [unwired: 6 in, 4 out]
          n117 = Format Into String(w318) -> (resulting string=w315:string)  [unwired: 3 in, 1 out]
          n118 = Equal?(x="localhost", y=w310) -> (x = y?=w313:bool)
          n119 = Select(t="", s=w313, f=w310) -> (s? t:f=w312:string)
          n120 = call <userlib>:"Set Cluster Element by Name__ogtk.vi"("Element Name (\"\": New Element Data Name)"=w315, "New Element Value"=w312, "Cluster"=w317) -> ("error out"=w321:errorcluster, "VCluster out"=w320:variant)  [unwired: 6 in, 1 out]
          n121 = Variant To Data(error in=w321, type=w317, Variant=w320) -> (data=w319:T1)  [unwired: 1 out]
          n122 = local write "Instrument Addresses"(w319) -> ()
        }
        n123 = call <vilib>:"Add State(s) to Queue__jki_lib_state_machine.vi"("State(s) in (\"\")"=w309) -> ("States Out"=w308:string)  [unwired: 14 in]
      }
      frame "---------- Instruments ----------" {
        # "Template Separator\n(You can make a copy of, or modify, this frame)"
        n124 = call <vilib>:"Add State(s) to Queue__jki_lib_state_machine.vi"("State(s) in (\"\")"=w326) -> ("States Out"=w325:string)  [unwired: 14 in]
      }
      frame "Instruments: Init Instruments" {
        # "#148 clear instrument classes after\nreading previously installed"
        # "Template Separator\n(You can make a copy of, or modify, this frame)"
        n125 = Unbundle By Name(w336) -> ("C.E."=w332:refnum<class "Control Experiment.lvclass">, "Installed Instruments"=w339:refnum<class "Instrument.lvclass">[], "Instrument Class Rings"=w340:refnum<vi>[])
        n126 = Bundle By Name(cluster=w332, "Instrument Classes"=T5 {"DAQ"=refnum, "Amplifier"=refnum, "Temperature"=refnum, "Magnet"=refnum, "Rotator"=refnum, "Level"=refnum, "Capacitance"=refnum, "Delay Line"=refnum, "Strain Cell"=refnum, "VNA"=refnum, "Source"=refnum}) -> (w331:refnum<class "Control Experiment.lvclass">)
        n127 = call <userlib>:"Get Cluster Element Names__ogtk.vi"("error in (no error)"=w328, "Cluster"="Instrument Addresses") -> ("error out"=w327:errorcluster, "Element Names"=w330:string[])  [unwired: 8 in]
        n128 = for {
          tunnel: "Instrument Addresses" -> [w348]
          tunnel: w340 -> [w355] mode=indexing
          shift-right: [w358] -> w334
          shift-left: w331 -> [w359]
          tunnel: w327 -> [w349]
          tunnel: w339 -> [w357]
          tunnel: [w356] -> w335 mode=indexing
          tunnel: w330 -> [w350] mode=indexing
          n129 = property class="Ring"(reference=w355) -> ("RingText.Text"=w351:string, "Label.Text"=w354:string)  [unwired: 1 in, 2 out]
          n130 = call <userlib>:"Get Cluster Element by Name__ogtk.vi"("error in (no error)"=w349, "Element Name"=w350, "Cluster"=w348) -> ("error out"=w347:errorcluster, "VElement"=w346:variant)  [unwired: 6 in, 1 out]
          n131 = Variant To Data(error in=w347, type="", Variant=w346) -> (data=w344:string, error out=w343:errorcluster)
          n132 = Scan From String(input string=w354, default 1=Instrument_Types--enum."DAQ" ("Type")) -> (output 1=w353:T6)  [unwired: 3 in, 3 out]
          n133 = case shown="Default" w351 {
            selector: w351 -> [_ w377]
            tunnel: w344 -> [_ w375]
            tunnel: w359 -> [w365 w380]
            tunnel: [w364 w379] -> w358
            tunnel: w343 -> [w361 w376]
            tunnel: w357 -> [_ w374]
            tunnel: [w362 w378] -> w356
            tunnel: w353 -> [w360 w371]
            frame "" {
              n134 = call "Insert Instrument Class by Name.vi"("error in (no error)"=w361, "Type"=w360, "Instrument in"=refnum<class "Instrument.lvclass"> refnum, "Control Experiment in"=w365) -> ("error out"=w362:errorcluster, "Control Experiment out"=w364:refnum<class "Control Experiment.lvclass">)  [unwired: 4 in, 2 out]
            }
            frame Default {
              n135 = call "Find Class by Name.vi"("error in (no error)"=w376, "Name"=w377, "Installed Instruments"=w374) -> ("error out"=w372:errorcluster, "Instrument out"=w373:refnum<class "Instrument.lvclass">)  [unwired: 7 in]
              n136 = call <userlib>:"Write SMO Address.vi"("error in (no error)"=w372, "Address"=w375, "Instrument in"=w373) -> ("error out"=w367:errorcluster, "Instrument out"=w370:refnum<class "Instrument.lvclass">)  [unwired: 7 in]
              n137 = call "Set IsConfigured.vi"("error in (no error)"=w367, "IsConfigured?"=TRUE, "SMO"=w370) -> ("error out"=w366:errorcluster, "SMO out"=w369:refnum<class "Instrument.lvclass">)  [unwired: 7 in]
              n138 = call "Insert Instrument Class by Name.vi"("error in (no error)"=w366, "Type"=w371, "Instrument in"=w369, "Control Experiment in"=w380) -> ("error out"=w378:errorcluster, "Control Experiment out"=w379:refnum<class "Control Experiment.lvclass">)  [unwired: 4 in, 2 out]
            }
          }
        }
        n139 = Bundle By Name(cluster=w336, "C.E."=w334) -> (w337:T7)
        n140 = Merge Errors(w335) -> (w338:errorcluster)
        n141 = call <vilib>:"Add State(s) to Queue__jki_lib_state_machine.vi"("State(s) in (\"\")"=w342) -> ("States Out"=w341:string)  [unwired: 14 in]
      }
    }
  }
  n142 = Unbundle By Name(w6) -> ("C.E."=w4:refnum<class "Control Experiment.lvclass">)
  n143 = call "Control Experiment Class to JSON.vi"("error in (no error)"=w2, "Control Experiment in"=w4) -> ("error out"=→"error out":errorcluster, "Control Experiment out"=→"Control Experiment":refnum<class "Control Experiment.lvclass">)  [unwired: 7 in, 1 out]
